vi "lockin - replace AO Sweep Indicator.vi"(8 "error in (no error)":errorcluster, 10 "Channels: AO.Sweeping?":bool[](array[boolean]), 11 "Instrument.DAQ":refnum<class "Instrument.DAQ.lvclass">) -> (0 "error out":errorcluster, 3 "Instrument.DAQout":refnum<class "Instrument.DAQ.lvclass">)   [LabVIEW 2019, in "Instrument.DAQ.lvclass"]
uses:
  Instrument.DAQ.lvclass
  Instrument.DAQ.lvclass/Instrument.DAQ.ctl
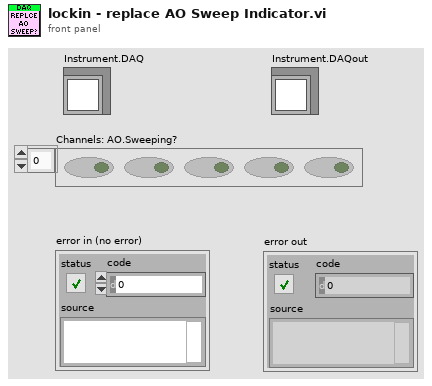
[diagram p1: front panel]
types:
  T1 = typedef "Instrument.DAQ.lvclass/AO.Channel--Cluster--Array.ctl" = T2[]
  T2 = typedef "Instrument.DAQ.lvclass/AO.Channel--Cluster.ctl" = cluster{"Enable?":bool, "Channel":i32, "Amplitude":dbl, "Offset":dbl, "Frequency":dbl, "Phase":dbl, "Function":T3, "Sweeping?":bool}
  T3 = typedef "Instrument.DAQ.lvclass/AO.Channel.Function--Enum.ctl" = enum16{"Sine", "Triangle", "Square"}
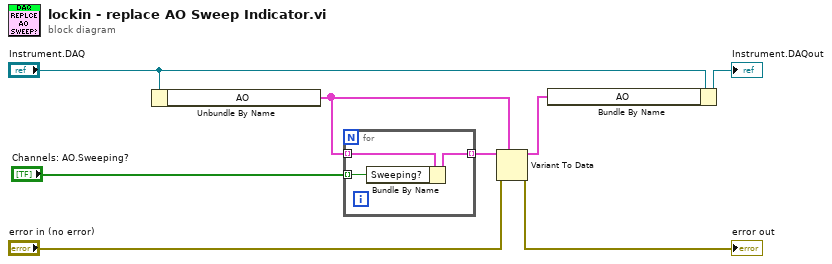
[diagram p0: block diagram]
diagram:
  n1 = Unbundle By Name("Instrument.DAQ") -> ("AO"=w5:T1)
  n2 = for {
    tunnel: w5 -> [w11] mode=indexing
    tunnel: "Channels: AO.Sweeping?" -> [w10] mode=indexing
    tunnel: [w9] -> w6 mode=indexing
    n3 = Bundle By Name(cluster=w11, "Sweeping?"=w10) -> (w9:T2)
  }
  n4 = Variant To Data(error in="error in (no error)", type=w5, Variant=w6) -> (data=w3:T1, error out=→"error out":errorcluster)
  n5 = Bundle By Name(cluster="Instrument.DAQ", "AO"=w3) -> (→"Instrument.DAQout":refnum<class "Instrument.DAQ.lvclass">)
